vi "GET.vi"(0 "url":string, 1 "response_len_out":i32, 5 "headers_json":string, 7 "timeout_ms":i32, 9 "handle_out":cluster{}, 11 "error in (no error)":errorcluster, 12 "status_out":u32) -> (3 "response_len_out out":i32, 4 "function return":i32, 10 "handle_out out":cluster{}, 14 "status_out out":u32, 15 "error out":errorcluster)   [LabVIEW 2020, in "reqwest-labview.lvlib"]
doc: "Performs an HTTP GET request and returns a handle and response length for use with http_read_response.\n\n\n\n\n\nint http_get(const char *url,\n const char *headers_json,\n int timeout_ms,\n unsigned long long *handle_out,\n int *response_len_out,\n unsigned int *status_out);"
uses:
  reqwest-labview.lvlib
  http_rs_labview.dll
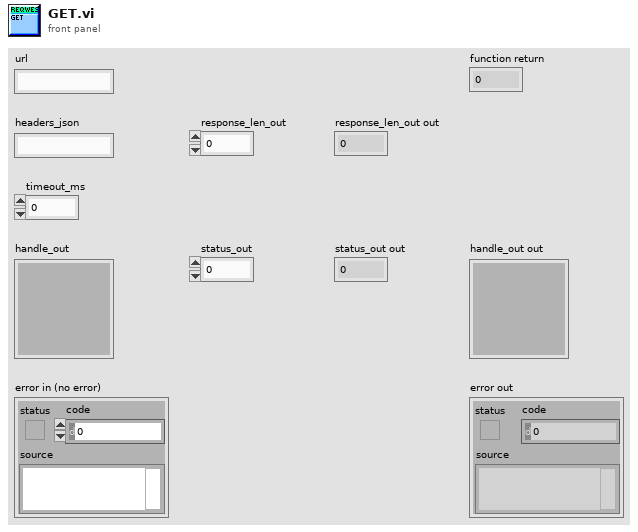
[diagram p1: front panel]
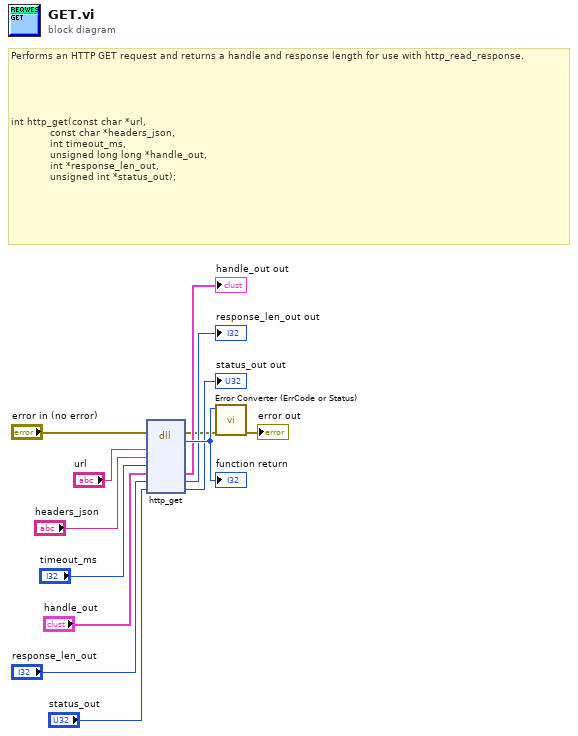
[diagram p0: block diagram]
diagram:
  # "Performs an HTTP GET request and returns a handle and response length for use with http_read_response.\n\n\n\n\n\nint http_get(const char *url,\n             const char *headers_json,\n             int timeout_ms,\n             unsigned long long *handle_out,\n             int *response_len_out,\n             unsigned int *status_out);"
  n1 = dll-call lib="C:/code/reqwest-labview/lv-src/shared-library/http_rs_labview.*" fn="http_get"(error in="error in (no error)", "url"="url", "headers_json"="headers_json", "timeout_ms"="timeout_ms", "handle_out"="handle_out", "response_len_out"="response_len_out", "status_out"="status_out") -> (error out=w2:errorcluster, w13:i32, "handle_out"=→"handle_out out":cluster{}, "response_len_out"=→"response_len_out out":i32, "status_out"=→"status_out out":u32)  [unwired: 5 in, 1 out]
  "function return" <- w13
  n2 = call "Error Converter (ErrCode or Status).vi"("error in (no error)"=w2, "error code"=w13) -> ("error out"=→"error out":errorcluster)  [unwired: 9 in]
